vi "Deney-Tek.vi"(1 "f unit":enum16{"mHz", "Hz", "kHz", "MHz", "GHz"}(ring)=enum."kHz", 5 "Frekans":i32(slide)=1 caption="Amplitude(V)" step=1 scale=0.0..100.0, 7 "Amplitude(V)":i32(slide)=20 scale=0.0..20.0, 9 "Teta Aralık":dbl=1.0) -> (6 "Real Matrix":T2)   [LabVIEW 2016]
uses:
  xcontrol/Start Button.xctl
  <vilib>/silver_ctls/ArrayMatrixCluster/Real Matrix NI_Silver.ctl
  <vilib>/Instr/_visa.llb/VISA Configure Serial Port (Instr).vi
  <instrlib>/Tektronix TDS 200 1000 2000 Series/Public/Data/Read (Single Waveform).vi
  <instrlib>/Tektronix TDS 200 1000 2000 Series/Tektronix TDS 200 1000 2000 Series.lvlib
panel:
  in  "Kaydet":path
  in  "Vert Range":dbl=5.0
  in  "polar attributes":T1={"maximum"=0.0, "minimum"=0.0, "clip to min"=FALSE, "log?(F)"=FALSE, "grid color"=12369084, "plot color"=16711680, "fmt and prec"={"format"=enum."Decimal", "precision"=2}, "visible section"=8} {"minimum" format="%0.2f"; "maximum" format="%0.2f"}
  out "XY Graph":cluster{i32[], "Real Matrix":dbl[]}(graph)={[0, 1, 2, 3, 4, 5, 6, 7, 8, 9, 10, 11, 12, 13, 14, 15, 16, 17, 18, 19, 20, 21, 22, 23, 24, 25, 26, 27, 28, 29, 30, 31, 32, 33, 34, 35, 36, 37, 38, 39, 40, 41, 42, 43, 44, 45, 46, 47, 48, 49, 50, 51, 52, 53, 54, 55, 56, 57, 58, 59, 60, 61, 62, 63, 64, 65, 66, 67, 68, 69, 70, 71, 72, 73, 74, 75, 76, 77, 78, 79, 80, 81, 82, 83, 84, 85, 86, 87, 88, 89, 90, 91, 92, 93, 94, 95, 96, 97, 98, 99, 100, 101, 102, 103, 104, 105, 106, 107, 108, 109, 110, 111, 112, 113, 114, 115, 116, 117, 118, 119, 120, 121, 122, 123, 124, 125, 126, 127, 128, 129, 130, 131, 132, 133, 134, 135, 136, 137, 138, 139, 140, 141, 142, 143, 144, 145, 146, 147, 148, 149, 150, 151, 152, 153, 154, 155, 156, 157, 158, 159, 160, 161, 162, 163, 164, 165, 166, 167, 168, 169, 170, 171, 172, 173, 174, 175, 176, 177, 178, 179, 180, 181, 182, 183, 184, 185, 186, 187, 188, 189, 190, 191, 192, 193, 194, 195, 196, 197, 198, 199, 200, 201, 202, 203, 204, 205, 206, 207, 208, 209, 210, 211, 212, 213, 214, 215, 216, 217, 218, 219, 220, 221, 222, 223, 224, 225, 226, 227, 228, 229, 230, 231, 232, 233, 234, 235, 236, 237, 238, 239, 240, 241, 242, 243, 244, 245, 246, 247, 248, 249, 250, 251, 252, 253, 254, 255, 256, 257, 258, 259, 260, 261, 262, 263, 264, 265, 266, 267, 268, 269, 270, 271, 272, 273, 274, 275, 276, 277, 278, 279, 280, 281, 282, 283, 284, 285, 286, 287, 288, 289, 290, 291, 292, 293, 294, 295, 296, 297, 298, 299, 300, 301, 302, 303, 304, 305, 306, 307, 308, 309, 310, 311, 312, 313, 314, 315, 316, 317, 318, 319, 320, 321, 322, 323, 324, 325, 326, 327, 328, 329, 330, 331, 332, 333, 334, 335, 336, 337, 338, 339, 340, 341, 342, 343, 344, 345, 346, 347, 348, 349, 350, 351, 352, 353, 354, 355, 356, 357, 358, 359], "Real Matrix"=[0.9370031393948146, 0.9385822794442714, 0.9381595180469032, 0.9389424923514267, 0.9371533285966223, 0.9342242421913879, 0.932194270415822, 0.9300204378030607, 0.9290440201922925, 0.9289530517332032, 0.9223086756666579, 0.9228351306884618, 0.9187688893108418, 0.9146225033320707, 0.9100200974541847, 0.908139888057528, 0.9030534887922861, 0.898997669863152, 0.8951920865335309, 0.8929155096221717, 0.8855171395548834, 0.8797330251136399, 0.8769104295358776, 0.870476812307048, 0.86276476671897, 0.8566850796594069, 0.8566360768337532, 0.8462794247142226, 0.8374941309273293, 0.8369997046033226, 0.8281464055071197, 0.8187398040083811, 0.8060006325138056, 0.8092615855757969, 0.7973546190632261, 0.7851638030510856, 0.7851812584636614, 0.7726850998604786, 0.7604304095486201, 0.7479771898348085, 0.7480387192185103, 0.7347201285474034, 0.7213854701826544, 0.7211040876268797, 0.706700842636502, 0.6896797668599796, 0.6700423025049215, 0.6701850137730759, 0.6581793856336107, 0.6369811278675201, 0.6215416809098601, 0.6212184513228259, 0.6024261144227047, 0.5807899031497097, 0.5836355674233913, 0.5592954646195468, 0.5394975779777519, 0.5199933982975492, 0.5197800807617362, 0.4959769528660494, 0.4749001200878623, 0.47697711626775424, 0.45099375157409743, 0.42970107402574953, 0.40739922103169074, 0.4055743931740193, 0.3817125133116575, 0.3564283820988305, 0.35754432346836046, 0.33109058635440136, 0.3093758545259001, 0.28257428703365306, 0.28248369721823924, 0.25600571934059135, 0.22939194680669336, 0.20204502546130332, 0.20191776754404267, 0.17691434918817767, 0.14989442785770093, 0.1497226271231765, 0.12418052078353856, 0.09563779663324827, 0.06929674806223038, 0.0694461222142385, 0.050752809600000004, 0.0482185632, 0.0504360288, 0.05523299519999999, 0.051363744, 0.04972668160481873, 0.053118227423022336, 0.07663290611758837, 0.10302654492278743, 0.10466492072213189, 0.12979834646751384, 0.156535582005932, 0.17823123786964046, 0.178188659340451, 0.2038083278925693, 0.22910113836972498, 0.2529326450787837, 0.2558280306549739, 0.27799087802857464, 0.3042037269187879, 0.30196626985110997, 0.3234995226985903, 0.3460732272260306, 0.36804602077200554, 0.3662460965611319, 0.3873137130311451, 0.40660818576777685, 0.4066109220004359, 0.4264808932079273, 0.4467382790515051, 0.46697495907784387, 0.46736108886866823, 0.48358797675807585, 0.5024984599668256, 0.5022574002447926, 0.5207339721501684, 0.5349811032719749, 0.553564645441777, 0.5514998902167627, 0.5663290160726488, 0.5818607673359145, 0.5962335231185176, 0.5965150490601955, 0.609326856423681, 0.624789759279714, 0.6224707159596415, 0.6377634864613746, 0.6483490316619233, 0.6601251609190342, 0.6581549106755359, 0.6701528883881218, 0.6803235365888548, 0.6800318512387401, 0.6899465697282554, 0.6993073138846948, 0.7067686412810904, 0.7065160755170176, 0.7147576719218692, 0.721793006133611, 0.7245919911080682, 0.7317544423452285, 0.7391236524225395, 0.7444583727436654, 0.7463221123464996, 0.7512647935914657, 0.759624839476617, 0.7626956274820573, 0.7640388703550797, 0.7680294509115264, 0.7728170866494378, 0.7713838334400189, 0.7764198969538892, 0.7824202731891579, 0.7867873529895001, 0.7847655654678767, 0.7917848766643406, 0.7925041352276947, 0.7944618890785811, 0.7977678150086287, 0.8006088408872721, 0.8026878171119477, 0.801750853154459, 0.805125853540143, 0.8099565331330503, 0.8070334413167708, 0.8082144579968511, 0.8109890609208251, 0.8137790559131551, 0.8139481741898383, 0.8148736867916107, 0.8163709868257303, 0.8177671804579336, 0.8188317767007313, 0.8173773849079543, 0.8171066352598378, 0.8192099656004997, 0.8193734773242711, 0.8193156625457974, 0.8194469278048362, 0.81882439735427, 0.8182885923437136, 0.8199971808786137, 0.8173175511471595, 0.8186834005480608, 0.81570993096097, 0.8161998736674545, 0.816374245024886, 0.8142584767759518, 0.8103335204610163, 0.8125474430516593, 0.8097572460709764, 0.8062817682035537, 0.804799847888472, 0.805726372771465, 0.8033930374594235, 0.799116576295398, 0.7939634451855606, 0.7946035301692257, 0.7905147754880846, 0.7870463231809799, 0.7861286759906899, 0.7828359362433486, 0.777541197841438, 0.7715052825734517, 0.7746972093809169, 0.7670895165196091, 0.7610733617470923, 0.7621113503351767, 0.7558379761864003, 0.7484625098594726, 0.7413752277113825, 0.7429490726044513, 0.73254720909472, 0.7246638526701885, 0.7256154595865563, 0.7174790598874013, 0.7077499780635859, 0.6987684517228394, 0.6992939982430001, 0.6870037940505923, 0.6764330859905998, 0.6644617430756895, 0.6657665954894562, 0.6512276770072912, 0.6397522157635255, 0.6398081188675872, 0.6253563882046895, 0.6113515135301804, 0.5976136718904548, 0.5952938027222472, 0.5795634294626828, 0.5637619105707777, 0.5625326026655076, 0.5461964297873336, 0.5287408208809915, 0.5115988789637952, 0.5099040694346822, 0.4906833462363496, 0.47272351455674355, 0.47187952667157207, 0.4523187712448592, 0.43139966903417043, 0.4097129622281879, 0.4104748985591283, 0.38886845143259036, 0.36797535472367093, 0.3431920731404687, 0.34494541730602457, 0.3219220461117111, 0.29716970860392317, 0.299119939156717, 0.2722505717182291, 0.24621627432674184, 0.21884553690362216, 0.22000235667820736, 0.19388470978973804, 0.16775975223470477, 0.16623275948599864, 0.1414765107759229, 0.1115351687442453, 0.08091115672798996, 0.08044643969902882, 0.05379983563678931, 0.055074604799999996, 0.0535585824, 0.0504360288, 0.0484674624, 0.0500513664, 0.05061704639999999, 0.07504189023849646, 0.10590097723638604, 0.13607394058040714, 0.13603994299356906, 0.16653398679562104, 0.19358242279733318, 0.19269299064774045, 0.22165820614021536, 0.24911752279555346, 0.2815668274240308, 0.2807729882472099, 0.3074800301975281, 0.33537877334028954, 0.33652331812606273, 0.361528164192581, 0.3883233097019497, 0.4147850928233051, 0.4157185775329378, 0.43993803824583266, 0.4630787437994681, 0.4647517224527514, 0.48951878370106156, 0.5122764927061004, 0.5346587646699439, 0.5375497485376848, 0.5598890888011707, 0.5813482395304662, 0.6019839150799321, 0.6022232379321389, 0.6232475227827783, 0.6409545542817486, 0.6422199400822581, 0.6641568054359103, 0.680004484824984, 0.6979127673725541, 0.699326603942441, 0.713405031592295, 0.7298158004770064, 0.7317800637659748, 0.7438835614277066, 0.7578298653560421, 0.7719326316046573, 0.7751095532427384, 0.7868108008819472, 0.7997674895680243, 0.7973934773102693, 0.8106350060863692, 0.8224753258516199, 0.8332466125572839, 0.8338355123544913, 0.8427811338545471, 0.8556515559749304, 0.864230307828579, 0.8630555565715788, 0.8711503413412749, 0.8807143543997566, 0.8797043393305185, 0.8879500126846566, 0.8955968627205879, 0.9000693587337563, 0.902176807266521, 0.9063232821527024, 0.9135101846718223, 0.9134358741567673, 0.9181813071512747, 0.9240211689827604, 0.9268169395289589, 0.9268055537616221, 0.9311845154784945, 0.9325672550229543, 0.9349935822115826, 0.9350912698075731, 0.9384416167257359, 0.9415353309777609, 0.9401291229209694, 0.943434110357225, 0.9442186817358811, 0.9453347459699804, 0.9456708560410467, 0.9446042341255825, 0.9461950828066158, 0.9465262450107378, 0.9452934838609071, 0.9459219000959679, 0.9425092257978079, 0.9444714190281827, 0.9444582170638792]}
  out "Polar Plot":picture
  out "OSC ERR":bool=TRUE
  out "Out Com":string="x"
  out "İlk Ayar":bool=TRUE
  out "Waveform Data":waveform(dbl)(graph)={"t0"=timestamp(-0.0024999999999999467 s since 1904-01-01), "dt"=2e-06, "Y"=array[2500 elements]}
  in  "Osiloskop Portu":refnum<visa-resource-name>="USB0::0x0699::0x0363::C102985::INSTR"
  in  "Start Button":dbl(xcontrol)
  in  "Reset Dafault":bool
  in  "Teta":u32(slide) scale=0.0..360.0
  in  "Sinyal Jeneratörü Portu":refnum<visa-resource-name>="COM4"
  in  "OUTPUT":bool=TRUE caption="Output"
  in  "cmdOrjin":bool
  in  "cmdStop":bool
  in  "Motor Sürücü Portu":refnum<visa-resource-name>="COM5"
  # "R-O Tarayıcı ile Bilgisayar Kontrollü Halka Anten Radyasyon Paterni Ölçüm Düzeneği Geliştirilmesi"
  # "Teta"
  # "Frekans"
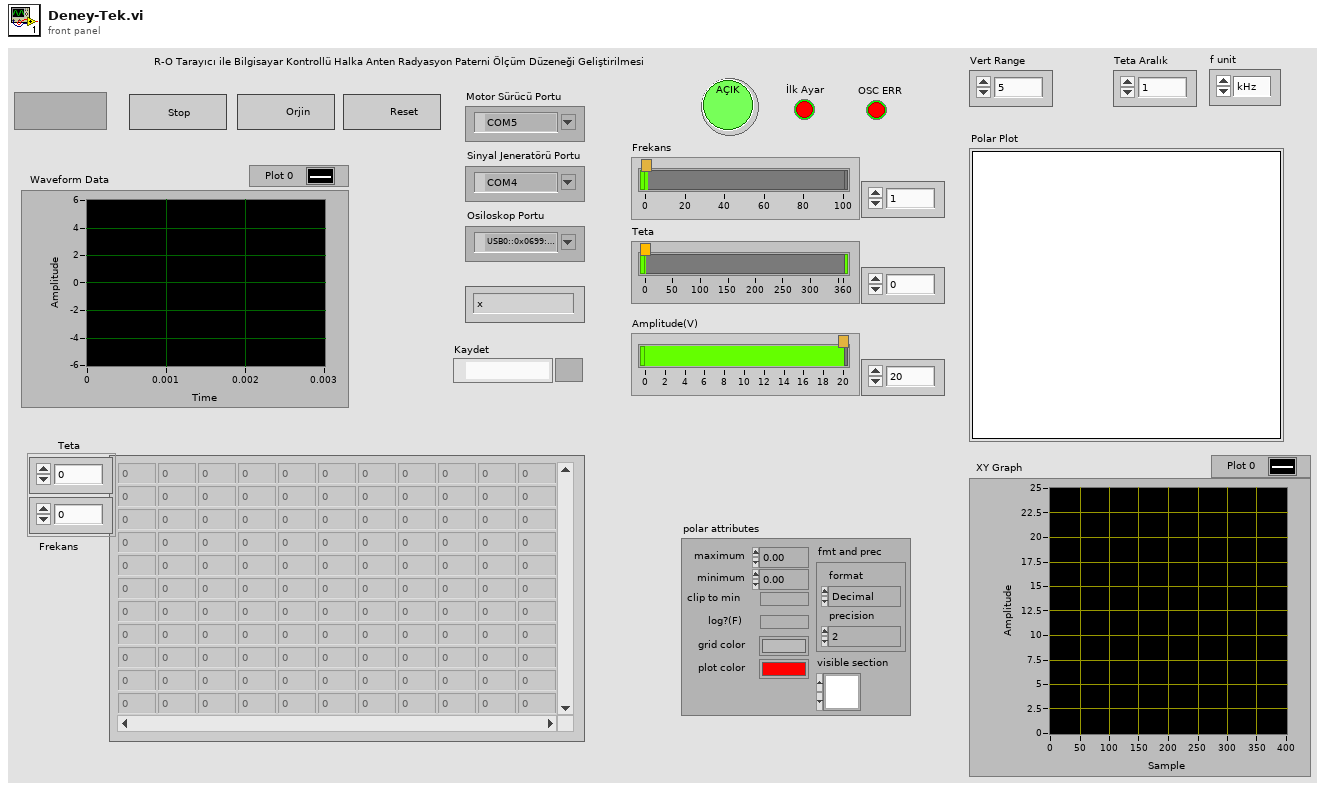
[diagram p1: front panel]
types:
  T1 = cluster{"maximum":dbl, "minimum":dbl, "clip to min":bool, "log?(F)":bool, "grid color":u32, "plot color":u32, "fmt and prec":cluster{"format":enum8{"Decimal", "Scientific", "Engineering", "Binary", "Octal", "Hex"}, "precision":u8}, "visible section":u16}
  T2 = typedef "Real Matrix NI_Silver.ctl" = dbl[][]
  T3 = cluster{"Baud Rate":u32, "Parity":u16, "Stop Bits":u16, "Flow Control":u16}
  T4 = typedef "NI_Matrix.lvlib/RealMatrix.ctl" = dbl[][]
  T5 = typedef "LVBoundsTypeDef.ctl" = cluster{"Width":u32, "Height":u32}
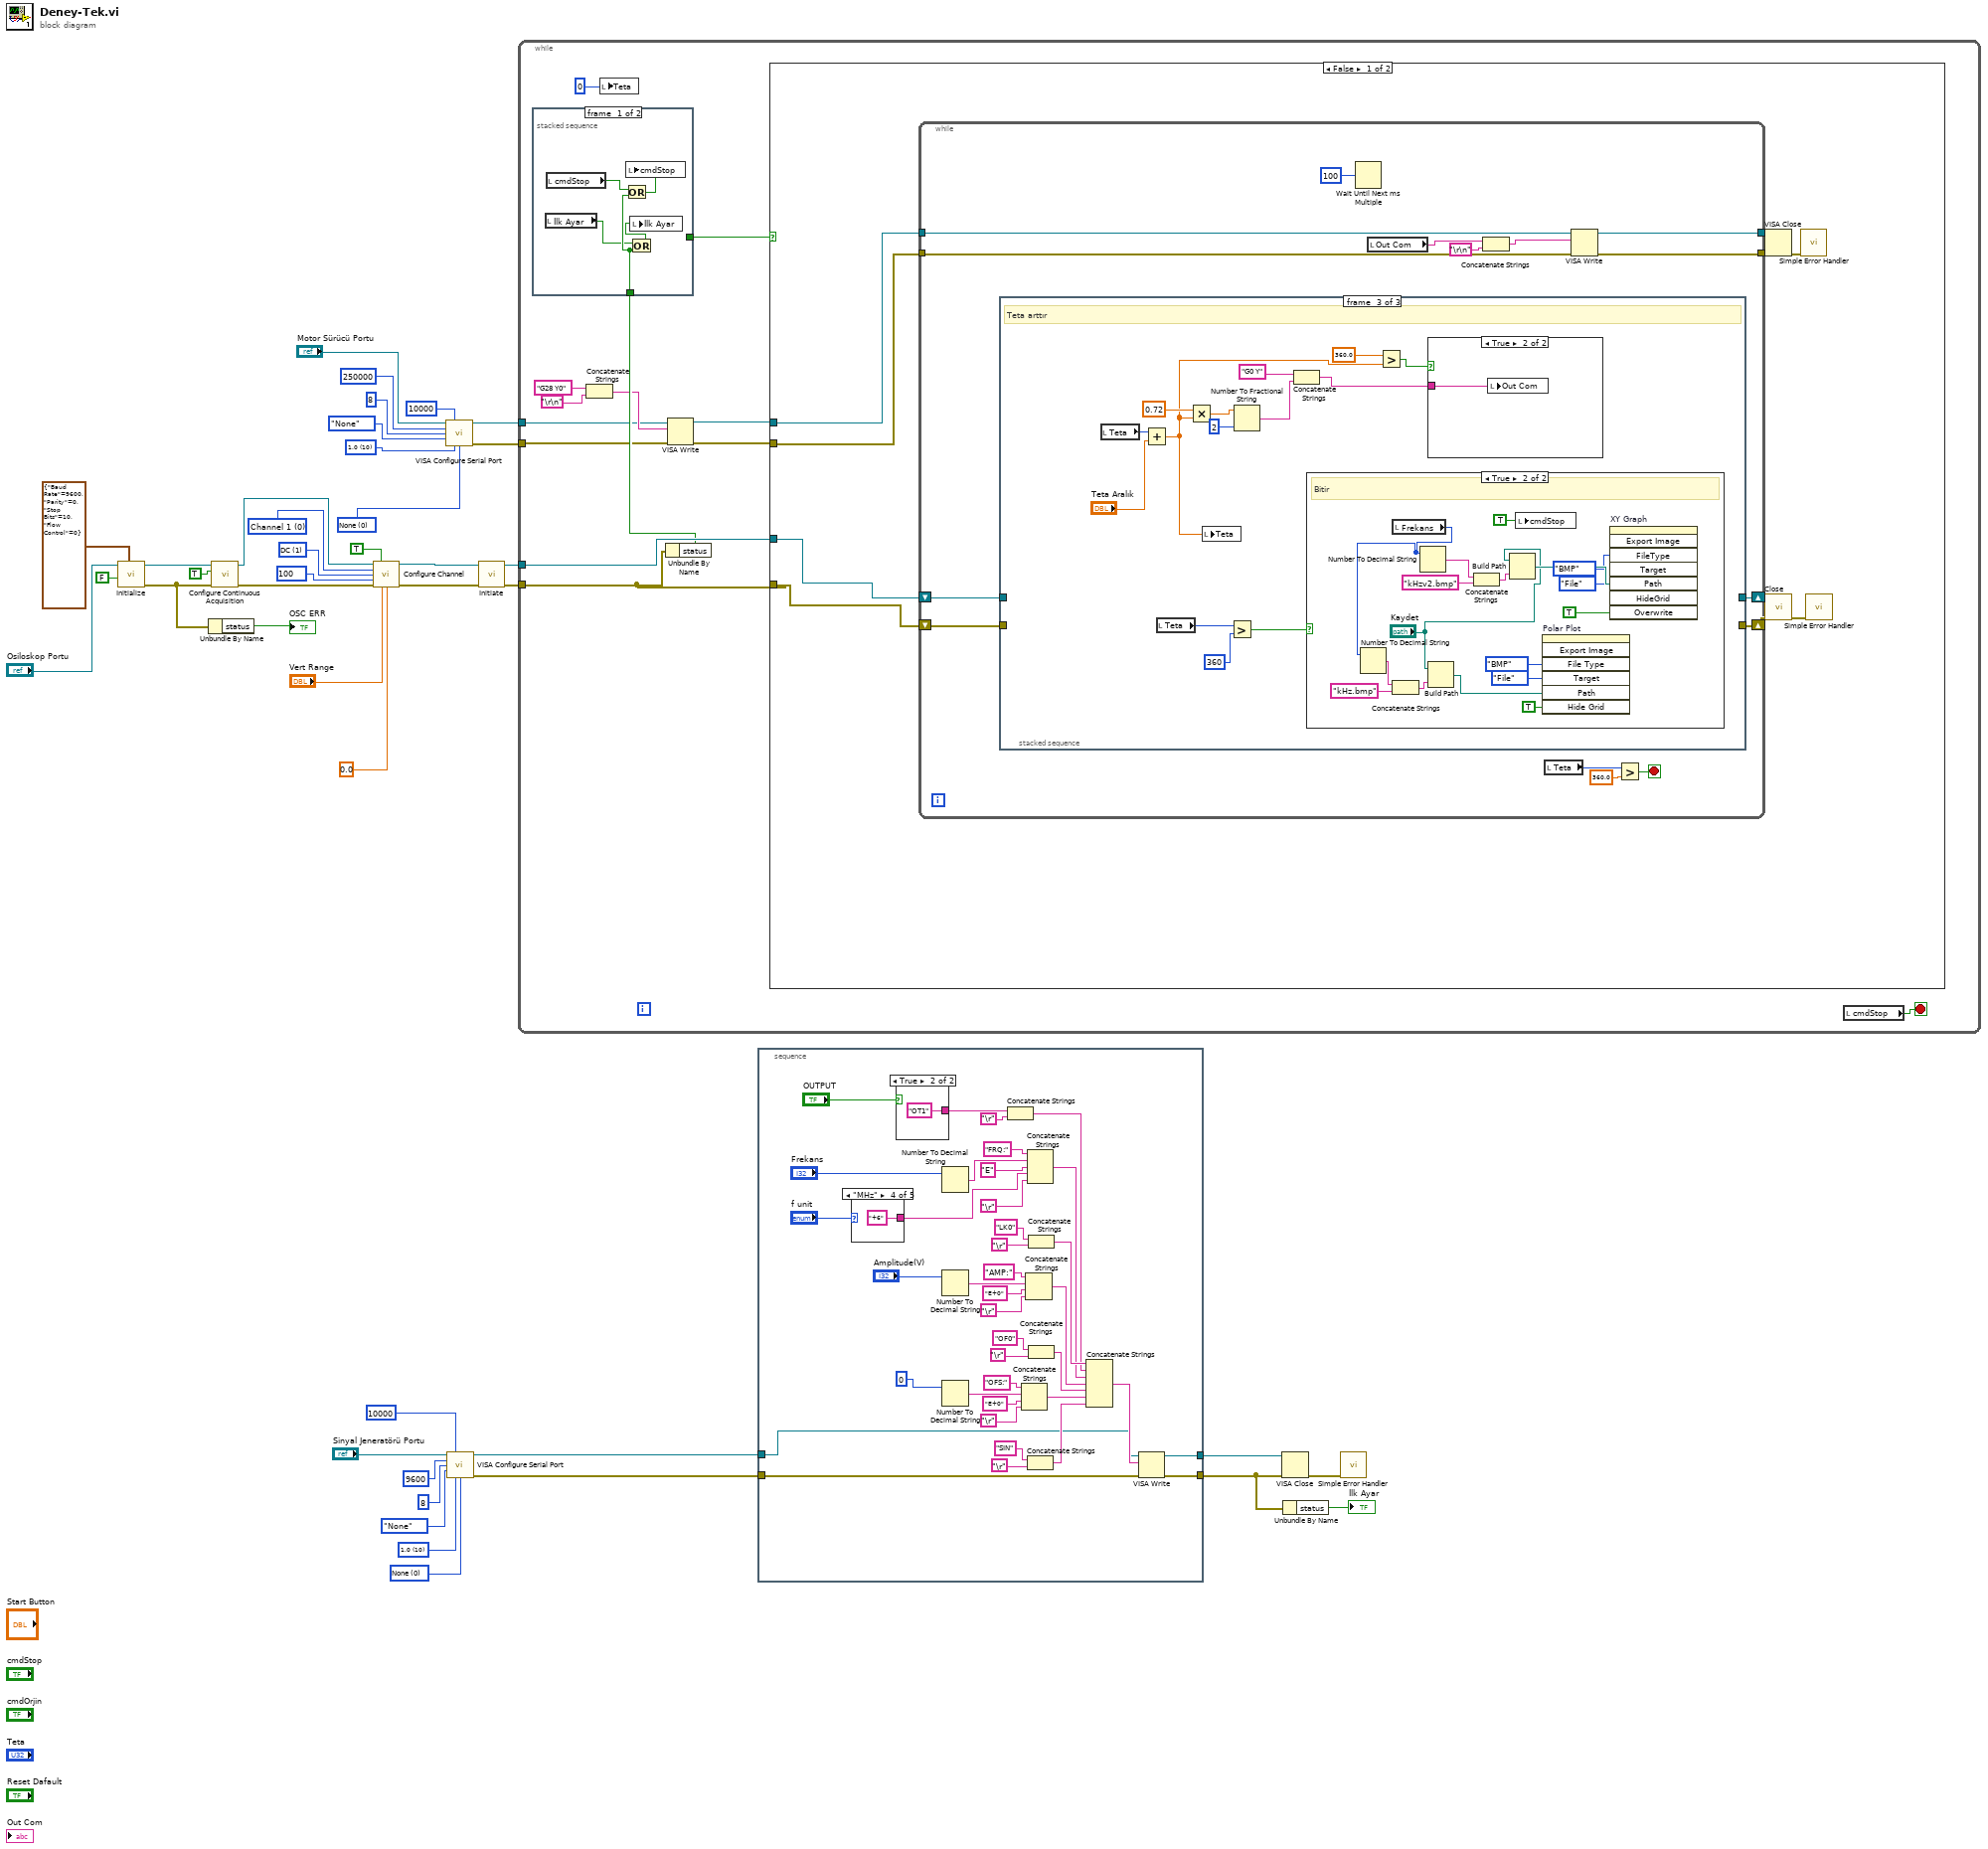
[diagram p0: block diagram]
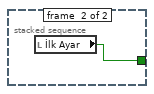
[diagram p2: hidden frame]
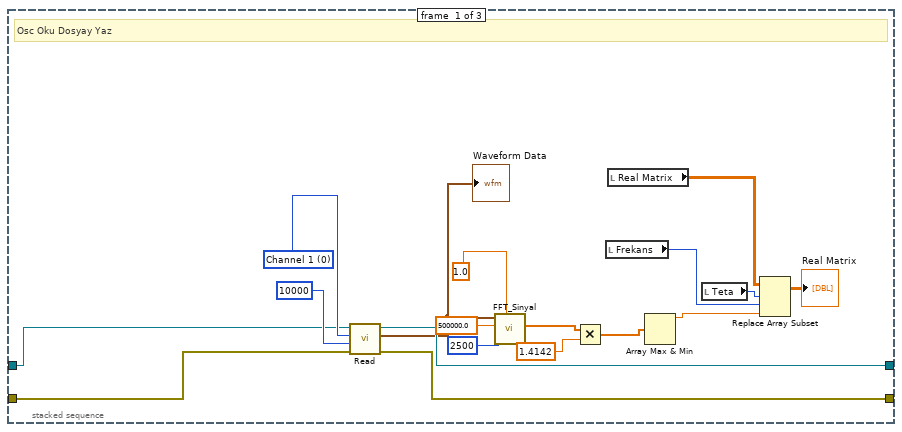
[diagram p3: hidden frame]
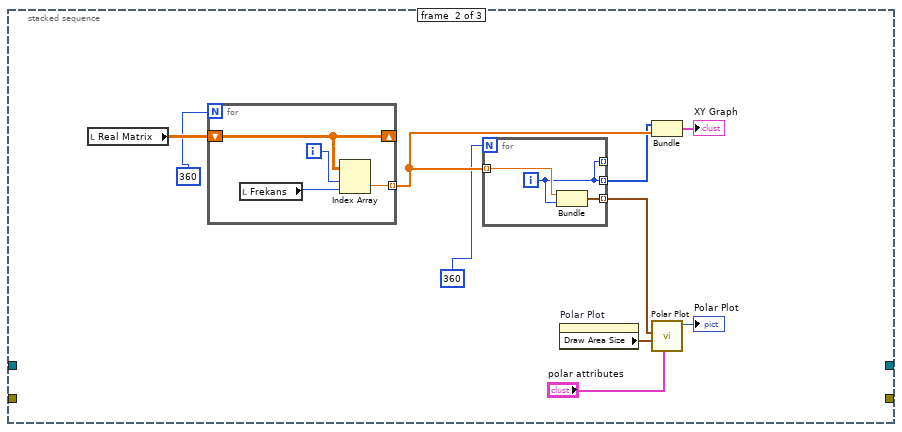
[diagram p4: hidden frame]
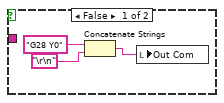
[diagram p5: hidden frame]
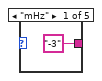
[diagram p8: hidden frame]
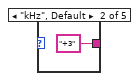
[diagram p9: hidden frame]
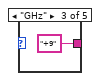
[diagram p10: hidden frame]
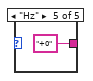
[diagram p11: hidden frame]
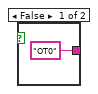
[diagram p12: hidden frame]
diagram:
  w15 = 1 items=["AC", "DC", "Ground"] ("Vertical Coupling (1: DC)")
  w16 = 0 items=["Channel 1", "Channel 2", "Channel 3", "Channel 4", "Math", "Reference A", "Reference B", "Reference C", "Reference D"] ("Channel (0: Channel 1)")
  w18 = 100 items=["1"=1, "10"=10, "20"=20, "50"=50, "100"=100, "500"=500, "1000"=1000] ("Probe Attenuation (10: 10X)")
  w34 = u16 0 items=["None", "XON/XOFF", "RTS/CTS", "XON/XOFF & RTS/CTS", "DTR/DSR", "XON/XOFF & DTR/DSR"] ("flow control (0:none)")
  w33 = u16 10 items=["1.0"=10, "1.5"=15, "2.0"=20] ("stop bits (10: 1 bit)")
  w35 = u16 0 items=["None", "XON/XOFF", "RTS/CTS", "XON/XOFF & RTS/CTS", "DTR/DSR", "XON/XOFF & DTR/DSR"] ("flow control (0:none)")
  w36 = u16 10 items=["1.0"=10, "1.5"=15, "2.0"=20] ("stop bits (10: 1 bit)")
  n1 = call <instrlib>:"Initialize.vi"("Serial Configuration"=T3 {"Baud Rate"=9600, "Parity"=0, "Stop Bits"=10, "Flow Control"=0} ("Osiloskop Config"), "Reset? (T: Yes)"=FALSE, "VISA resource name"="Osiloskop Portu") -> ("error out"=w4:errorcluster, "VISA resource name out"=w5:refnum<visa-resource-name>)  [unwired: 2 in, 5 out]
  n2 = Unbundle By Name(w4) -> ("status"=→"OSC ERR":bool)
  n3 = call <instrlib>:"Configure Continuous Acquisition.vi"("error in (no error)"=w4, "Enable Continuous Acquisition Mode (True)"=TRUE, "VISA resource name"=w5) -> ("error out"=w19:errorcluster, "VISA resource name out"=w22:refnum<visa-resource-name>)  [unwired: 7 out]
  n4 = call <instrlib>:"Configure Channel.vi"("VISA resource name"=w22, "Enable Channel (True)"=TRUE, "Channel (0: Channel 1)"=w16, "Vertical Coupling (1: DC)"=w15, "Probe Attenuation (10: 10X)"=w18, "error in (no error)"=w19, "Vertical Range (10.0 V/div)"="Vert Range", "Vertical Offset (0.0 divs)"=0.0) -> ("VISA resource name out"=w21:refnum<visa-resource-name>, "error out"=w20:errorcluster)  [unwired: 6 in]
  n5 = call-poly "VISA Configure Serial Port"("VISA resource name"="Motor Sürücü Portu", "timeout (10sec)"=u32 10000, "baud rate (9600)"=u32 250000, "data bits (8)"=u16 8, "parity (0:none)"=enum16{"None", "Odd", "Even", "Mark", "Space"}."None", "stop bits (10: 1 bit)"=w36, "flow control (0:none)"=w35) -> ("VISA resource name out"=w8:refnum<visa-resource-name>, "error out"=w7:errorcluster)  [unwired: 7 in]
  n6 = call-poly "VISA Configure Serial Port"("VISA resource name"="Sinyal Jeneratörü Portu", "timeout (10sec)"=u32 10000, "baud rate (9600)"=u32 9600, "data bits (8)"=u16 8, "parity (0:none)"=enum16{"None", "Odd", "Even", "Mark", "Space"}."None", "stop bits (10: 1 bit)"=w33, "flow control (0:none)"=w34) -> ("VISA resource name out"=w13:refnum<visa-resource-name>, "error out"=w12:errorcluster)  [unwired: 7 in]
  n7 = call <instrlib>:"Initiate.vi"("error in (no error)"=w20, "VISA resource name"=w21) -> ("error out"=w23:errorcluster, "VISA resource name out"=w24:refnum<visa-resource-name>)  [unwired: 8 out]
  n8 = while {
    tunnel: w24 -> [w54]
    tunnel: w23 -> [w52]
    tunnel: w8 -> [w46]
    tunnel: w7 -> [w43]
    stop <- w53 stop-if-true
    n9 = Concatenate Strings("G28 Y0" ("string"), "\r\n") -> (w47:string)
    n10 = local write "Teta"(u32 0 ("Teta")) -> ()
    n11 = Unbundle By Name(w52) -> ("status"=w51:bool)
    n12 = stacked-sequence {
      tunnel: w51 -> [w56 _]
      tunnel: [_ w60] -> w50
      frame #0 {
        n13 = local read "İlk Ayar"() -> (w55:bool)
        n14 = local read "cmdStop"() -> (w58:bool)
        n15 = Or(x=w58, y=w56) -> (x .or. y?=w59:bool)
        n16 = local write "cmdStop"(w59) -> ()
        n17 = Or(x=w55, y=w56) -> (x .or. y?=w57:bool)
        n18 = local write "İlk Ayar"(w57) -> ()
      }
      frame #1 {
        n19 = local read "İlk Ayar"() -> (w60:bool)
      }
    }
    n20 = VISA Write(VISA resource name=w46, write buffer=w47, error in (no error)=w43) -> (VISA resource name out=w45:refnum<visa-resource-name>, error out=w44:errorcluster)  [unwired: 1 out]
    n21 = case shown="False" w50 {
      tunnel: w54 -> [w62 _]
      tunnel: w52 -> [w61 _]
      tunnel: w45 -> [w68 _]
      tunnel: w44 -> [w67 _]
      frame False {
        n22 = while {
          shift-right: [w83] -> w70
          shift-left: w62 -> [w85]
          shift-right: [w82] -> w69
          shift-left: w61 -> [w84]
          tunnel: w68 -> [w77]
          tunnel: w67 -> [w76]
          tunnel: [w75] -> w65
          tunnel: [w74] -> w64
          stop <- w73 stop-if-true
          n23 = stacked-sequence {
            tunnel: w85 -> [w95 _ _]
            tunnel: w84 -> [w94 _ _]
            tunnel: [w101 _ _] -> w82
            tunnel: [w100 _ _] -> w83
            frame #0 {
              w102 = u16 0 items=["Channel 1", "Channel 2", "Channel 3", "Channel 4", "Math", "Reference A", "Reference B", "Reference C", "Reference D"] ("Channel B (1: Channel 2)")
              # "Osc Oku Dosyay Yaz"
              n24 = call-poly <instrlib>:"Read.vi"("error in (no error)"=w94, "Timeout (10000 ms)"=u32 10000 ("Timeout (10000 ms) 2"), "Source (0: Channel 1)"=w102, "VISA resource name"=w95) -> ("error out"=w101:errorcluster, "Waveform Data"=w93:waveform(dbl), "VISA resource name out"=w100:refnum<visa-resource-name>)  [unwired: 5 out]
              "Waveform Data" <- w93
              n25 = call "FFT_Sinyal.vi"("Oran"=1.0, "Number of Sample"=2500, "Sampling Frequency"=500000.0, "Sinyal"=w93) -> ("Sinyal Genlik"=w89:dbl[])  [unwired: 2 in, 3 out]
              n26 = Multiply(x=w89, y=1.4142) -> (x*y=w87:dbl[])
              n27 = local read "Frekans"() -> (w97:i32)
              n28 = local read "Real Matrix"() -> (w98:T2)
              n29 = Array Max & Min(array=w87) -> (max value=w86:dbl)  [unwired: 3 out]
              n30 = local read "Teta"() -> (w96:u32)
              n31 = Replace Array Subset ("Set Matrix Elements")(array=w98, new element=w86, index (row)=w96, index (col)=w97) -> (→"Real Matrix":T4)
            }
            frame #1 {
              n32 = local read "Real Matrix"() -> (w113:T2)
              n33 = for {
                N: 360 -> [_]
                shift-right: [w119] -> _
                shift-left: w113 -> [w119]
                tunnel: [w120] -> w112 mode=indexing
                i -> [w118]
                n34 = local read "Frekans"() -> (w117:i32)
                n35 = Index Array(array=w119, index (row)=w118, index (col)=w117) -> (element=w120:dbl)
              }
              n36 = for {
                N: 360 -> [_]
                tunnel: [w115] -> w110 mode=indexing
                tunnel: [w114] -> _ mode=indexing
                tunnel: [w114] -> w106 mode=indexing
                tunnel: w112 -> [w116] mode=indexing
                i -> [w114]
                n37 = Bundle("Numeric"=w116, w114) -> (w115:cluster{"Numeric":dbl, i32})  [unwired: 1 in]
              }
              n38 = property on="Polar Plot" class="Pict"() -> ("Draw Area Size"=w109:T5)  [unwired: 2 in, 2 out]
              n39 = Bundle(w106, w112) -> (→"XY Graph":cluster{i32[], dbl[]})  [unwired: 1 in]
              n40 = call <vilib>:"Polar Plot.vi"("polar attributes"="polar attributes", "dimensions (w,h)"=w109, "data array [mag, phase (deg)]"=w110) -> ("new picture"=→"Polar Plot":picture)  [unwired: 8 in]
            }
            frame #2 {
              # "Teta arttır"
              n41 = local read "Teta"() -> (w134:u32)
              n42 = Add(x=w134, y="Teta Aralık") -> (x+y=w124:dbl)
              n43 = local read "Teta"() -> (w133:u32)
              n44 = Multiply(x=0.72, y=w124) -> (x*y=w126:dbl)
              n45 = local write "Teta"(w124) -> ()
              n46 = Greater?(x=w133, y=360) -> (0:w131:bool)
              n47 = Number To Fractional String(number=w126, precision (6)=i16 2) -> (F-format string=w127:string)  [unwired: 2 in]
              n48 = Concatenate Strings("G0 Y" ("Out Com"), w127) -> (w121:string)
              n49 = case shown="True" w131 {
                frame False {
                }
                frame True {
                  # "Bitir"
                  n50 = local read "Frekans"() -> (w139:i32)
                  n51 = Number To Decimal String(number=w139) -> (decimal integer string=w144:string)  [unwired: 1 in]
                  n52 = Concatenate Strings(w144, "kHz.bmp" ("string")) -> (w142:string)
                  n53 = Number To Decimal String(number=w139) -> (decimal integer string=w154:string)  [unwired: 1 in]
                  n54 = Build Path(base path="Kaydet", name or relative path=w142) -> (appended path=w141:path)
                  n55 = Concatenate Strings(w154, "kHzv2.bmp" ("string")) -> (w152:string)
                  n56 = Build Path(base path="Kaydet", name or relative path=w152) -> (appended path=w151:path)
                  n57 = local write "cmdStop"(TRUE ("cmdStop")) -> ()
                  n58 = invoke on="Polar Plot" class="Pict" method="Export Image"("File Type"=enum32{"BMP", "EPS", "EMF", "PICT"}."BMP", "Target"=enum32{"File", "Clipboard"}."File", "Path"=w141, "Hide Grid"=TRUE ("Always Overwrite")) -> ()  [unwired: 3 in, 7 out]
                  n59 = invoke on="XY Graph" class="XYGraph (strict)" method="Export Image"("FileType"=enum32{"BMP", "EPS", "EMF", "PICT"}."BMP" ("File Type"), "Target"=enum32{"File", "Clipboard"}."File", "Path"=w151, "Overwrite"=TRUE ("Always Overwrite")) -> ()  [unwired: 4 in, 8 out]
                }
              }
              n60 = Greater?(x=360.0, y=w124) -> (0:w122:bool)
              n61 = case shown="True" w122 {
                tunnel: w121 -> [_ w138]
                frame False {
                  n62 = Concatenate Strings("G28 Y0" ("string"), "\r\n") -> (w135:string)
                  n63 = local write "Out Com"(w135) -> ()
                }
                frame True {
                  n64 = local write "Out Com"(w138) -> ()
                }
              }
            }
          }
          n65 = Wait Until Next ms Multiple(millisecond multiple=u32 100) -> ()  [unwired: 1 out]
          n66 = local read "Out Com"() -> (w80:string)
          n67 = Concatenate Strings(w80, "\r\n") -> (w79:string)
          n68 = local read "Teta"() -> (w71:u32)
          n69 = VISA Write(VISA resource name=w77, write buffer=w79, error in (no error)=w76) -> (VISA resource name out=w75:refnum<visa-resource-name>, error out=w74:errorcluster)  [unwired: 1 out]
          n70 = Greater?(x=w71, y=360.0) -> (0:w73:bool)
        }
        n71 = VISA Close(VISA resource name=w65, error in (no error)=w64) -> (error out=w66:errorcluster)
        n72 = call <instrlib>:"Close.vi"("error in (no error)"=w69, "VISA resource name"=w70) -> ("error out"=w63:errorcluster)  [unwired: 9 in]
        n73 = call <vilib>:"Simple Error Handler.vi"("error in (no error)"=w66) -> ()  [unwired: 4 in, 5 out]
        n74 = call <vilib>:"Simple Error Handler.vi"("error in (no error)"=w63) -> ()  [unwired: 4 in, 5 out]
      }
      frame True {
      }
    }
    n75 = local read "cmdStop"() -> (w53:bool)
  }
  n76 = stacked-sequence {
    tunnel: w13 -> [w162]
    tunnel: w12 -> [w161]
    tunnel: [w160] -> w11
    tunnel: [w159] -> w6
    frame #0 {
      n77 = case shown="\"MHz\"" "f unit" {
        tunnel: ["-3" "+3" "+9" "+6" "+0"] -> w158
        frame "mHz" {
        }
        frame "kHz", Default {
        }
        frame "GHz" {
        }
        frame "MHz" {
        }
        frame "Hz" {
        }
      }
      n78 = case shown="True" "OUTPUT" {
        tunnel: ["OT0" "OT1"] -> w189
        frame False {
        }
        frame True {
        }
      }
      n79 = Number To Decimal String(number="Frekans") -> (decimal integer string=w184:string)  [unwired: 1 in]
      n80 = Number To Decimal String(number="Amplitude(V)") -> (decimal integer string=w178:string)  [unwired: 1 in]
      n81 = Number To Decimal String(number=0) -> (decimal integer string=w171:string)  [unwired: 1 in]
      n82 = Concatenate Strings(w189, "\r") -> (w186:string)
      n83 = Concatenate Strings("OFS:", w171, "E+0", "\r") -> (w170:string)
      n84 = Concatenate Strings("AMP:", w178, "E+0", "\r") -> (w177:string)
      n85 = Concatenate Strings("FRQ:", w184, "E", w158, "\r") -> (w183:string)
      n86 = Concatenate Strings("SIN", "\r") -> (w169:string)
      n87 = Concatenate Strings("LK0", "\r") -> (w187:string)
      n88 = Concatenate Strings("OF0", "\r") -> (w174:string)
      n89 = Concatenate Strings(w187, w186, w183, w177, w174, w170, w169) -> (w163:string)
      n90 = VISA Write(VISA resource name=w162, write buffer=w163, error in (no error)=w161) -> (VISA resource name out=w160:refnum<visa-resource-name>, error out=w159:errorcluster)  [unwired: 1 out]
    }
  }
  n91 = VISA Close(VISA resource name=w11, error in (no error)=w6) -> (error out=w10:errorcluster)
  n92 = Unbundle By Name(w6) -> ("status"=→"İlk Ayar":bool)
  n93 = call <vilib>:"Simple Error Handler.vi"("error in (no error)"=w10) -> ()  [unwired: 4 in, 5 out]
